vi "Calculate Average RGB From Histogram.vi"(11 "Histograms (R=row 0, G=row 1, B=row 2)":u32[][](array[numeric])) -> (3 "Color":u32(colorbox))   [LabVIEW 2015]
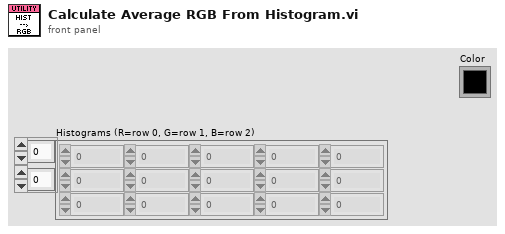
[diagram p1: front panel]
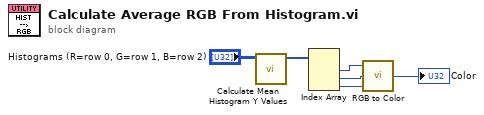
[diagram p0: block diagram]
diagram:
  n1 = call "Calculate Mean Histogram Y Values.vi"("Histograms"="Histograms (R=row 0, G=row 1, B=row 2)") -> ("Mean Row Values"=w1:u8[])  [unwired: 10 in]
  n2 = Index Array(array=w1) -> (element #1=w5:u8, element #2=w4:u8, element #3=w3:u8)  [unwired: 3 in]
  n3 = call <vilib>:"RGB to Color.vi"("B"=w3, "G"=w4, "R"=w5) -> ("Color"=→"Color":u32)
